vi "Relaxed Minimum.vi"() -> ()   [LabVIEW 2016]
panel:
  in  "d rel":dbl[](array[numeric])=[10.0, 1.0, 0.0, 0.1, 1.0, 1.0, 1.0, 1.0, 1.0, 1.0] format="%_4g"
  out "XY Graph":cluster{dbl[], dbl[]}(graph)={[0.5, 0.51, 0.52, 0.53, 0.54, 0.55, 0.56, 0.5700000000000001, 0.5800000000000001, 0.5900000000000001, 0.6000000000000001, 0.6100000000000001, 0.6200000000000001, 0.6300000000000001, 0.6400000000000001, 0.6500000000000001, 0.6600000000000001, 0.6700000000000002, 0.6800000000000002, 0.6900000000000002, 0.7000000000000002, 0.7100000000000002, 0.7200000000000002, 0.7300000000000002, 0.7400000000000002, 0.7500000000000002, 0.7600000000000002, 0.7700000000000002, 0.7800000000000002, 0.7900000000000003, 0.8000000000000003, 0.8100000000000003, 0.8200000000000003, 0.8300000000000003, 0.8400000000000003, 0.8500000000000003, 0.8600000000000003, 0.8700000000000003, 0.8800000000000003, 0.8900000000000003, 0.9000000000000004, 0.9100000000000004, 0.9200000000000004, 0.9300000000000004, 0.9400000000000004, 0.9500000000000004, 0.9600000000000004, 0.9700000000000004, 0.9800000000000004, 0.9900000000000004, 1.0000000000000004, 1.0100000000000005, 1.0200000000000005, 1.0300000000000005, 1.0400000000000005, 1.0500000000000005, 1.0600000000000005, 1.0700000000000005, 1.0800000000000005, 1.0900000000000005, 1.1000000000000005, 1.1100000000000005, 1.1200000000000006, 1.1300000000000006, 1.1400000000000006, 1.1500000000000006, 1.1600000000000006, 1.1700000000000006, 1.1800000000000006, 1.1900000000000006, 1.2000000000000006, 1.2100000000000006, 1.2200000000000006, 1.2300000000000006, 1.2400000000000007, 1.2500000000000007, 1.2600000000000007, 1.2700000000000007, 1.2800000000000007, 1.2900000000000007, 1.3000000000000007, 1.3100000000000007, 1.3200000000000007, 1.3300000000000007, 1.3400000000000007, 1.3500000000000008, 1.3600000000000008, 1.3700000000000008, 1.3800000000000008, 1.3900000000000008, 1.4000000000000008, 1.4100000000000008, 1.4200000000000008, 1.4300000000000008, 1.4400000000000008, 1.4500000000000008, 1.4600000000000009, 1.4700000000000009, 1.4800000000000009, 1.4900000000000009, 1.5000000000000009, 1.510000000000001, 1.520000000000001, 1.530000000000001, 1.540000000000001, 1.550000000000001, 1.560000000000001, 1.570000000000001, 1.580000000000001, 1.590000000000001, 1.600000000000001, 1.610000000000001, 1.620000000000001, 1.630000000000001, 1.640000000000001, 1.650000000000001, 1.660000000000001, 1.670000000000001, 1.680000000000001, 1.690000000000001, 1.700000000000001, 1.710000000000001, 1.720000000000001, 1.730000000000001, 1.740000000000001], [3.583015597634215, 3.583098611907087, 3.582768324570747, 3.57895668605634, 3.5787750586043243, 3.5718032265513147, 3.570143619460223, 3.569291553454106, 3.568411263570846, 3.5647116015520974, 3.564823562711806, 3.5622764146725157, 3.5618385391484026, 3.5598176526812098, 3.557805090088414, 3.555416093665239, 3.5545299955374956, 3.551121307446201, 3.546888901905601, 3.548008170571802, 3.5461331753426326, 3.5442530224549693, 3.5433394084126695, 3.5411299993329863, 3.5429707034749587, 3.5372946161745227, 3.53564685607615, 3.5327465070059945, 3.5295845207789003, 3.5278504885283937, 3.527827216987189, 3.521935750219405, 3.523141671980636, 3.521988435918996, 3.5198398207497905, 3.5195253327334606, 3.5166891529008253, 3.5151527025336105, 3.5159851360312087, 3.5143413468857942, 3.513910702837289, 3.512105598620847, 3.5110804939294336, 3.5109792700788294, 3.508378165257445, 3.5072636712390275, 3.5077232932101943, 3.5064102719095502, 3.505154982518819, 3.5064697719898525, 3.50344130470619, 3.5052106172960844, 3.503964737460309, 3.5037292529709863, 3.506551071737765, 3.501829954237062, 3.505105261630868, 3.5049212716480413, 3.5048090451617084, 3.5040998336662326, 3.5034972780416354, 3.504628547500542, 3.5033265940510434, 3.5018544832053875, 3.5038022554159336, 3.505809163560853, 3.5033197348691094, 3.504977223622723, 3.5061270051797813, 3.5034574531952827, 3.5051397881152844, 3.5060906567279364, 3.505848769405785, 3.5078908845171544, 3.5101983235733836, 3.510861046990855, 3.510074632619505, 3.5069172909990654, 3.513243638396676, 3.517200222074439, 3.5170774293103984, 3.5026444505227072, 3.5015426847449564, 3.502075649339976, 3.505932101439336, 3.512209486731778, 3.510238978684426, 3.5080925726646215, 3.510161791239988, 3.510665541811123, 3.5157063608288674, 3.5188654925077056, 3.518160364049693, 3.5205323206594445, 3.5250931636472944, 3.526170989527602, 3.5286704337919623, 3.5309888662465303, 3.532209060288528, 3.532428276962195, 3.5358868984843395, 3.539234355265955, 3.5376550280953314, 3.5353393868870913, 3.5395304392490377, 3.546602056284127, 3.546871968408636, 3.5479619509015117, 3.5549135935425564, 3.5522926688291108, 3.563848285549666, 3.5634588503698934, 3.567298943558519, 3.567718997106658, 3.5727551725106994, 3.57805408140336, 3.5806356925893916, 3.5823532349953076, 3.5880599237862203, 3.591401386441653, 3.59340707026726, 3.599487455890218, 3.603947315064133, 3.6055268473123827, 3.6113278470291506]}
  in  "dBc":dbl=0.01
  in  "Bc max":dbl=1.75
  in  "Bc min":dbl=0.5
  in  "Array In":dbl[](array[numeric])=[6.160000000000001, 0.5790000000000001, 0.962, 1.529145000000002, 0.19400000000000006, 0.36800000000000005, 0.43250000000000044, 0.23399999999999999, 0.05299999999999999, 3.5118302523269453] format="%_6g"
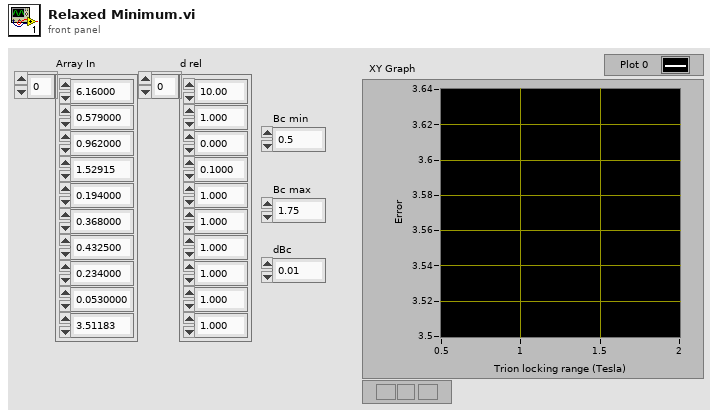
[diagram p1: front panel]
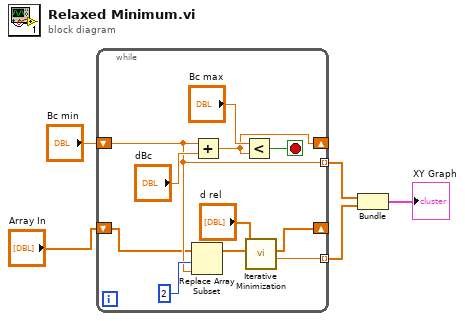
[diagram p0: block diagram]
diagram:
  n1 = while {
    shift-right: [w9] -> _
    shift-left: "Bc min" -> [w11]
    tunnel: [w11] -> w4 mode=indexing
    tunnel: [w10] -> w3 mode=indexing
    shift-right: [w7] -> _
    shift-left: "Array In" -> [w6]
    stop <- w12 stop-if-true
    n2 = Replace Array Subset(array=w6, new element=w11, index=2) -> (w16:dbl[])
    n3 = Add(x=w11, y="dBc") -> (x+y=w9:dbl)
    n4 = Less?(x="Bc max", y=w9) -> (x < y?=w12:bool)
    n5 = call "Iterative Minimization.vi"("d rel"="d rel", "Array In"=w16) -> ("Minima"=w10:dbl, "Array Out"=w7:dbl[])  [unwired: 8 in]
  }
  n6 = Bundle(w4, w3) -> (→"XY Graph":cluster{dbl[], dbl[]})  [unwired: 1 in]
